vi "Configure List Sweep.vi"(0 "VISA resource name":refnum<visa-resource-name>, 1 "Enable List Sweep (F: Disable)":bool, 2 "Sweep List Data":dbl[](array[numeric]), 3 "Sweep List Start Index (1)":i32=1, 5 "Channel (0: Channel 1)":i32(ring) items=["Channel 1", "Channel 2"], 9 "List Sweep Setting Mode (1: Voltage)":i32(ring)=1 items=["Current", "Voltage"], 11 "error in (no error)":errorcluster, 13 "Sweep List Data Mode (1: New List)":i32(ring)=1 items=["Append", "New List"]) -> (4 "VISA resource name out":refnum<visa-resource-name>, 15 "error out":errorcluster)   [LabVIEW 2020, in "Agilent B2900 Series.lvlib"]
doc: "Change settings for list sweep. \nThe list sweep function is effective for performing an arbitrary waveform output. The SMU can apply the waveform and measure voltage or current at each output value.\nUse Enable Output.vi to start outputting the value set by the Configure Source.vi\nUse Initiate.vi to perform the specified list sweep output and measurement."
uses:
  Agilent B2900 Series.lvlib
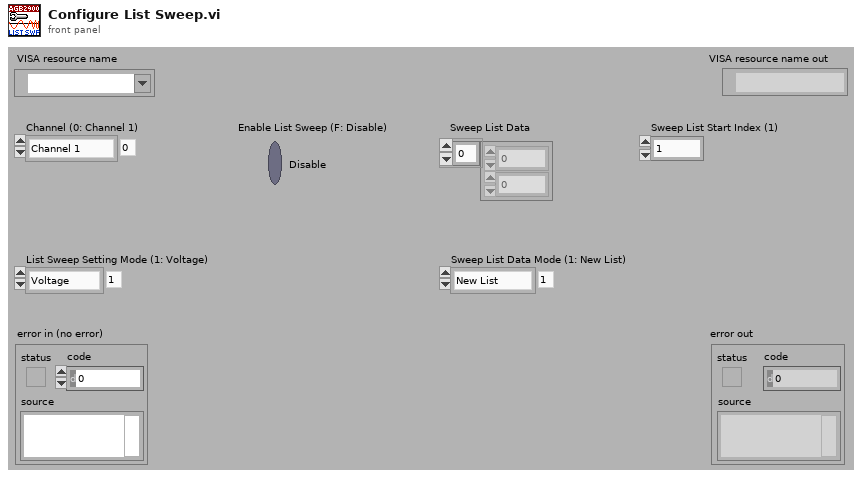
[diagram p1: front panel]
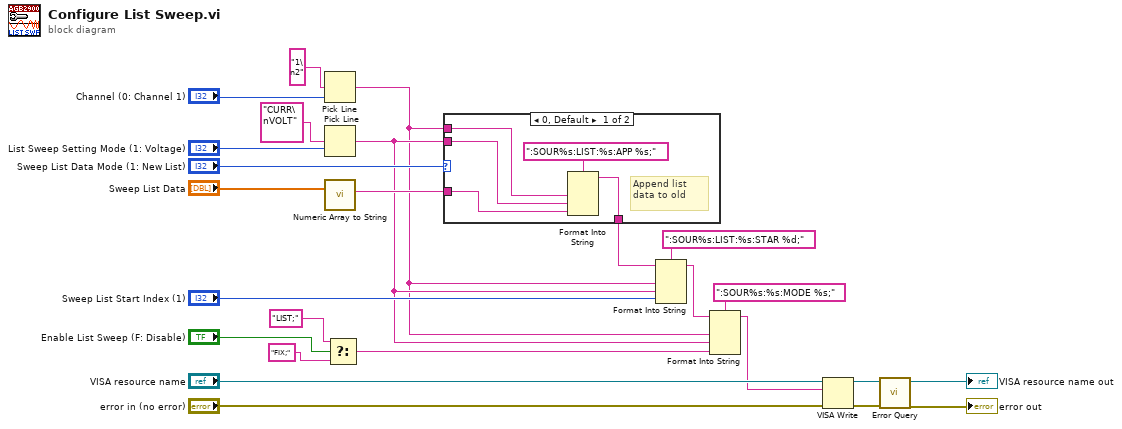
[diagram p0: block diagram]
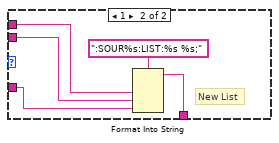
[diagram p2: hidden frame]
diagram:
  n1 = Pick Line(multi-line string="1\n2" ("string (\"\")"), line index="Channel (0: Channel 1)") -> (output string=w2:string)  [unwired: 1 in]
  n2 = Pick Line(multi-line string="CURR\nVOLT" ("string (\"\")"), line index="List Sweep Setting Mode (1: Voltage)") -> (output string=w6:string)  [unwired: 1 in]
  n3 = call "Numeric Array to String.vi"("List Data"="Sweep List Data") -> ("Result String"=w12:string)  [unwired: 10 in]
  n4 = Select(t="LIST;", s="Enable List Sweep (F: Disable)", f="FIX;") -> (s? t:f=w3:string)
  n5 = case shown="0, Default" "Sweep List Data Mode (1: New List)" {
    tunnel: w2 -> [w29 w34]
    tunnel: w6 -> [w28 w33]
    tunnel: w12 -> [w27 w32]
    tunnel: [w26 w31] -> w11
    frame 0, Default {
      # "Append list data to old"
      n6 = Format Into String(format string=":SOUR%s:LIST:%s:APP %s;", w29, w28, w27) -> (resulting string=w26:string)  [unwired: 2 in, 1 out]
    }
    frame 1 {
      # "New List"
      n7 = Format Into String(format string=":SOUR%s:LIST:%s %s;", w34, w33, w32) -> (resulting string=w31:string)  [unwired: 2 in, 1 out]
    }
  }
  n8 = Format Into String(format string=":SOUR%s:LIST:%s:STAR %d;", initial string=w11, w2, w6, "Sweep List Start Index (1)") -> (resulting string=w7:string)  [unwired: 1 in, 1 out]
  n9 = Format Into String(format string=":SOUR%s:%s:MODE %s;", initial string=w7, w2, w6, w3) -> (resulting string=w1:string)  [unwired: 1 in, 1 out]
  n10 = VISA Write(VISA resource name="VISA resource name", write buffer=w1, error in (no error)="error in (no error)") -> (VISA resource name out=w22:refnum<visa-resource-name>, error out=w21:errorcluster)  [unwired: 1 out]
  n11 = call "Error Query.vi"("error in (no error)"=w21, "VISA resource name"=w22) -> ("error out"=→"error out":errorcluster, "VISA resource name out"=→"VISA resource name out":refnum<visa-resource-name>)  [unwired: 6 in, 2 out]
